vi "Color Sensor V3 Update Color Match.vi"(10 "Color":cluster{"R":dbl, "G":dbl, "B":dbl}, 11 "Name":string) -> ()   [LabVIEW 2023]
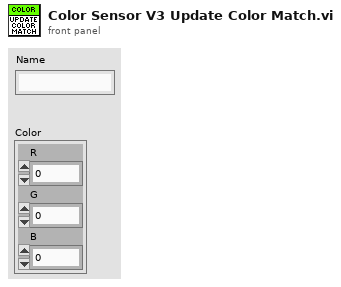
[diagram p1: front panel]
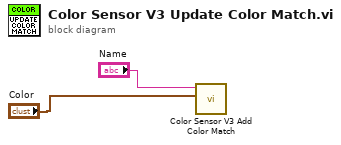
[diagram p0: block diagram]
diagram:
  n1 = call "Color Sensor V3 Add Color Match.vi"("Color"="Color", "Name"="Name") -> ()  [unwired: 10 in]
